vi "RTS Build Door Path Array.vi"(8 "Error In":errorcluster, 9 "Station":u8=1 min=1 max=8 step=1, 10 "Input":T1, 11 "Full Door Ops Path":path) -> (0 "Error Out":errorcluster, 2 "Output":T1)   [LabVIEW 2020]
uses:
  Type Definitions/RTS Test Pattern.ctl
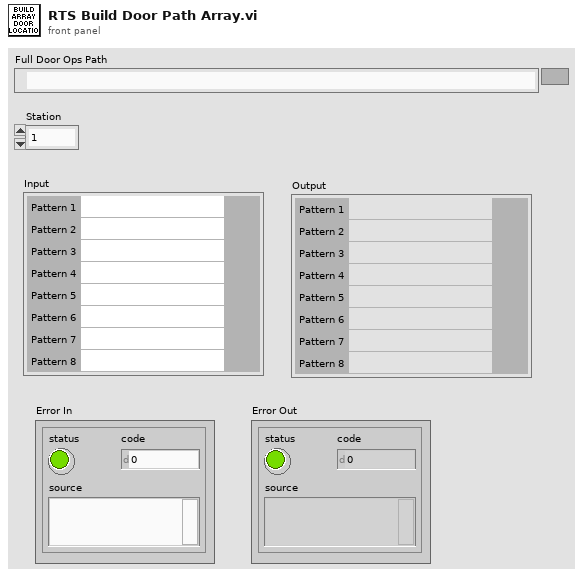
[diagram p1: front panel]
types:
  T1 = typedef "RTS Test Pattern.ctl" = cluster{" Pattern 1":path, "Pattern 2":path, "Pattern 3":path, "Pattern 4":path, "Pattern 5":path, "Pattern 6":path, "Pattern 7":path, "Pattern 8":path}
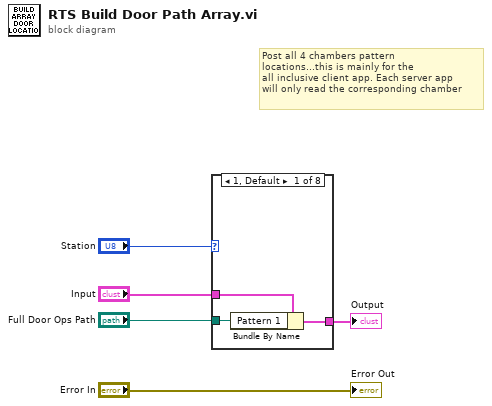
[diagram p0: block diagram]
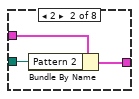
[diagram p2: hidden frame]
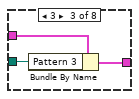
[diagram p3: hidden frame]
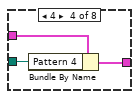
[diagram p4: hidden frame]
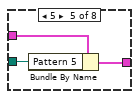
[diagram p5: hidden frame]
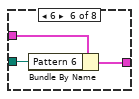
[diagram p6: hidden frame]
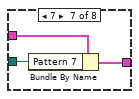
[diagram p7: hidden frame]
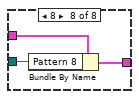
[diagram p8: hidden frame]
diagram:
  # "Post all 4 chambers pattern \nlocations...this is mainly for the \nall inclusive client app. Each server app\nwill only read the corresponding chamber"
  n1 = case shown="1, Default" "Station" {
    tunnel: "Input" -> [w8 w11 w14 w17 w20 w23 w26 w29]
    tunnel: [w7 w10 w13 w16 w19 w22 w25 w28] -> w1
    tunnel: "Full Door Ops Path" -> [w6 w9 w12 w15 w18 w21 w24 w27]
    frame 1, Default {
      n2 = Bundle By Name(cluster=w8, "Pattern 1"=w6) -> (w7:T1)
    }
    frame 2 {
      n3 = Bundle By Name(cluster=w11, "Pattern 2"=w9) -> (w10:T1)
    }
    frame 3 {
      n4 = Bundle By Name(cluster=w14, "Pattern 3"=w12) -> (w13:T1)
    }
    frame 4 {
      n5 = Bundle By Name(cluster=w17, "Pattern 4"=w15) -> (w16:T1)
    }
    frame 5 {
      n6 = Bundle By Name(cluster=w20, "Pattern 5"=w18) -> (w19:T1)
    }
    frame 6 {
      n7 = Bundle By Name(cluster=w23, "Pattern 6"=w21) -> (w22:T1)
    }
    frame 7 {
      n8 = Bundle By Name(cluster=w26, "Pattern 7"=w24) -> (w25:T1)
    }
    frame 8 {
      n9 = Bundle By Name(cluster=w29, "Pattern 8"=w27) -> (w28:T1)
    }
  }
  "Output" <- w1
  "Error Out" <- "Error In"
